vi "tank drive execute.vi"(0 "leftSpeed":dbl, 1 "rightSpeed":dbl, 2 "motorController":string, 4 "desiredDistanceLeft":dbl, 5 "desiredDistanceRight":dbl, 6 "driveMotors":string, 7 "leftMotor":string, 9 "rightMotor":string) -> ()   [LabVIEW 2019, in "Encoder Recorder.lvlib"]
uses:
  Encoder Recorder.lvlib
  <vilib>/Rock Robotics/WPI/Utilities/WPI_GetSetVariantRefNum.vi
  <vilib>/Rock Robotics/WPI/ThirdParty/Phoenix-LabVIEW/Motor Controller/Get/CTRE_Phoenix_MotorController_GetSelectedSensorData.vi
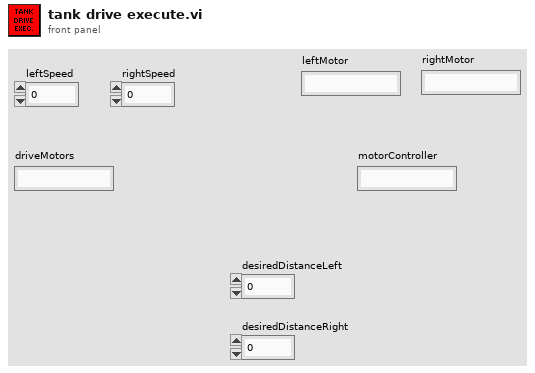
[diagram p1: front panel]
types:
  T1 = typedef "WPI_MotorControlDeviceRef.ctl" = cluster{"DeviceStatus":errorcluster, "Type":T2, "PWM":cluster{"PWM Channel":T3, "DeadBand":T4}, "CAN":cluster{"Device Number":u8, "SetOutput VI Ref":variant, "GetOutput VI Ref":variant, "Enable VI Ref":variant, "Disable VI Ref":variant, "Data":variant}, "Invert":bool, "DIO PWM":cluster{"PWM \"Enable\" Channel":T3, "DIOChannel":T5, "PWM Rate":dbl}}
  T2 = typedef "WPI_MotorControlType.ctl" = enum16{"PWM", "CAN", "DIO PWM"}
  T3 = typedef "FPGA_DIOPWMChannel.ctl" = enum8{"PWM 0", "PWM 1", "PWM 2", "PWM 3", "PWM 4", "PWM 5", "PWM 6", "PWM 7", "PWM 8", "PWM 9", "PWM MXP 0", "PWM MXP 1", "PWM MXP 2", "PWM MXP 3", "PWM MXP 4", "PWM MXP 5", "PWM MXP 6", "PWM MXP 7", "PWM MXP 8", "PWM MXP 9", "Invalid"}
  T4 = typedef "WPI_PWMDeadband.ctl" = cluster{"Name":string, "maxPositivePwm":i32, "minPositivePwm":i32, "centerPwm":i32, "maxNegativePwm":i32, "minNegativePwm":i32, "angularRange":u16}
  T5 = typedef "FPGA_DIOChannel.ctl" = enum8{"DIO 0", "DIO 1", "DIO 2", "DIO 3", "DIO 4", "DIO 5", "DIO 6", "DIO 7", "DIO 8", "DIO 9", "DIO MXP 0", "DIO MXP 1", "DIO MXP 2", "DIO MXP 3", "DIO MXP 4", "DIO MXP 5", "DIO MXP 6", "DIO MXP 7", "DIO MXP 8", "DIO MXP 9", "DIO MXP 10", "DIO MXP 11", "DIO MXP 12", "DIO MXP 13", "DIO MXP 14", "DIO MXP 15", "SPI Port CS1", "SPI Port CS2", "SPI Port CS3", "SPI Port MISO", "SPI Port MOSI", "Invalid"}
  T6 = typedef "WPI_RobotDriveDevRef.ctl" = cluster{"DevStatus":errorcluster, "Motors[]":T1[], "Square Inputs":bool, "Max Output":dbl}
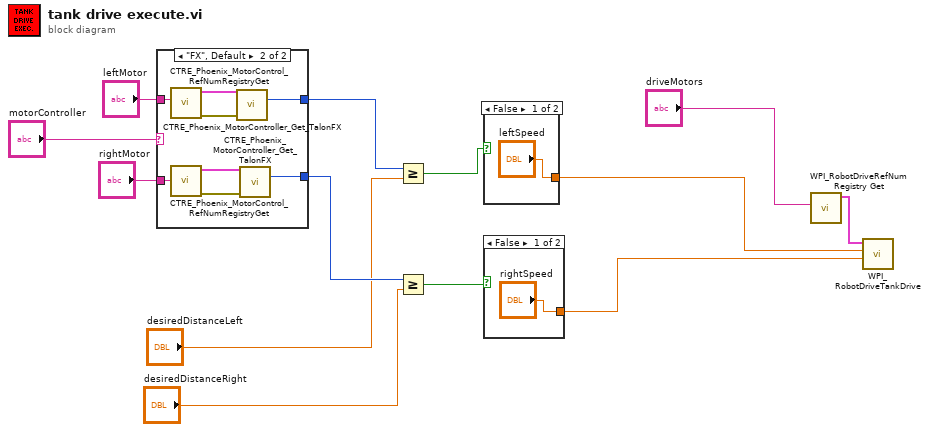
[diagram p0: block diagram]
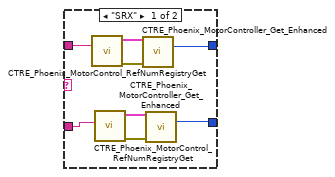
[diagram p2: hidden frame]
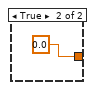
[diagram p3: hidden frame]
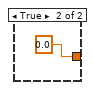
[diagram p4: hidden frame]
diagram:
  n1 = case shown="\"FX\", Default" "motorController" {
    tunnel: "leftMotor" -> [w21 w29]
    tunnel: [w18 w27] -> w6
    tunnel: "rightMotor" -> [w14 w25]
    tunnel: [w15 w24] -> w4
    frame "SRX" {
      n2 = call <vilib>:"CTRE_Phoenix_MotorControl_RefNumRegistryGet.vi"("refnum name"=w21) -> ("error out"=w19:errorcluster, "PhoenixMotorControlDevRef"=w20:T1)  [unwired: 9 in]
      n3 = call <vilib>:"CTRE_Phoenix_MotorControl_RefNumRegistryGet.vi"("refnum name"=w14) -> ("error out"=w16:errorcluster, "PhoenixMotorControlDevRef"=w17:T1)  [unwired: 9 in]
      n4 = call-poly <vilib>:"CTRE_Phoenix_MotorController_Get_Enhanced.vi"("PhoenixMotorControlDevRef"=w20, "error in"=w19) -> ("Position (Raw Sensor Units)"=w18:i32)  [unwired: 10 in, 3 out]
      n5 = call-poly <vilib>:"CTRE_Phoenix_MotorController_Get_Enhanced.vi"("PhoenixMotorControlDevRef"=w17, "error in"=w16) -> ("Position (Raw Sensor Units)"=w15:i32)  [unwired: 10 in, 3 out]
    }
    frame "FX", Default {
      n6 = call <vilib>:"CTRE_Phoenix_MotorControl_RefNumRegistryGet.vi"("refnum name"=w29) -> ("error out"=w23:errorcluster, "PhoenixMotorControlDevRef"=w28:T1)  [unwired: 9 in]
      n7 = call <vilib>:"CTRE_Phoenix_MotorControl_RefNumRegistryGet.vi"("refnum name"=w25) -> ("error out"=w22:errorcluster, "PhoenixMotorControlDevRef"=w26:T1)  [unwired: 9 in]
      n8 = call-poly <vilib>:"CTRE_Phoenix_MotorController_Get_TalonFX.vi"("PhoenixMotorControlDevRef"=w28, "error in"=w23) -> ("Position (Raw Sensor Units)"=w27:i32)  [unwired: 10 in, 3 out]
      n9 = call-poly <vilib>:"CTRE_Phoenix_MotorController_Get_TalonFX.vi"("PhoenixMotorControlDevRef"=w26, "error in"=w22) -> ("Position (Raw Sensor Units)"=w24:i32)  [unwired: 10 in, 3 out]
    }
  }
  n10 = Greater Or Equal?(x=w6, y="desiredDistanceLeft") -> (x >= y?=w10:bool)
  n11 = Greater Or Equal?(x=w4, y="desiredDistanceRight") -> (x >= y?=w8:bool)
  n12 = case shown="False" w10 {
    tunnel: ["leftSpeed" 0.0 ("leftSpeed")] -> w11
    frame False {
    }
    frame True {
    }
  }
  n13 = case shown="False" w8 {
    tunnel: ["rightSpeed" 0.0 ("leftSpeed")] -> w9
    frame False {
    }
    frame True {
    }
  }
  n14 = call <vilib>:"WPI_RobotDriveRefNum Registry Get.vi"("refnum name"="driveMotors") -> ("RobotDriveDevRef"=w12:T6)  [unwired: 9 in, 1 out]
  n15 = call <vilib>:"WPI_RobotDriveTankDrive.vi"("Right axis value"=w9, "Left axis value"=w11, "RobotDriveDevRef"=w12) -> ()  [unwired: 6 in, 3 out]
